vi "2 Think.vi"() -> ()   [LabVIEW 2011]
doc: "The Think VI performs the logic to determine which setpoints to send to the boat. Within the Think VI, a variety of systems take the boat information and output sail and rudder setpoints. The Think VI contains the arbiter VI which contains the logic used to determine which setpoints will ultimately be sent to the boat.\n\nWithin the Think VI, 5 systems are considered, in order of inherent priority:\n-Manual Override\n-Don't Flip\n-Staying out of/getting out of Irons\n-Getting to the goal\n-Default (such that there is always something being sent to the boat)"
uses:
  2 Globals/2 Global.vi
  2 Typedefs/sail setpt.ctl
  2 Typedefs/rudder angle.ctl
  2 Typedefs/setpoints to boat.ctl
  2 Typedefs/setpoints to arbiter.ctl
panel:
  out "Setpoints \nBefore Smoothing":T1
  out "Default Setpoints":T4
  out "Get to Goal Setpoints":T4
  out "Get Out of Irons Setpoints":T4
  out "Don't Flip Setpoints":T4
  out "Override Setpoints":T4
  out "Final Setpoints":T1
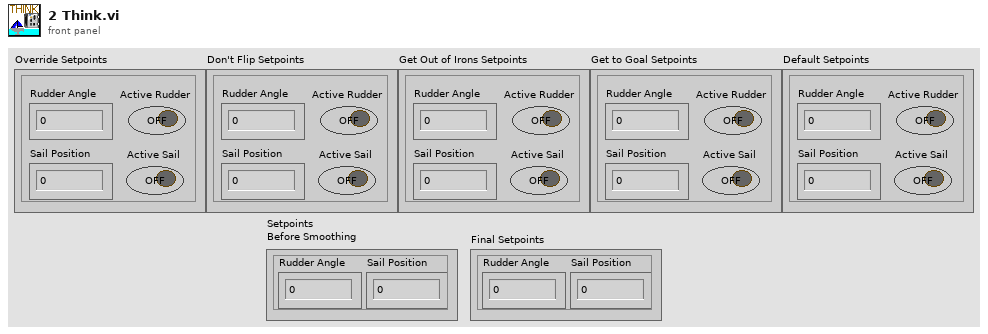
[diagram p1: front panel]
types:
  T1 = typedef "setpoints to boat.ctl" = cluster{"Sail Position":T2, "Rudder Angle":T3}
  T2 = typedef "sail setpt.ctl" = dbl
  T3 = typedef "rudder angle.ctl" = dbl
  T4 = typedef "setpoints to arbiter.ctl" = cluster{"Rudder Angle":dbl, "Sail Position":dbl, "Active Rudder":bool, "Active Sail":bool}
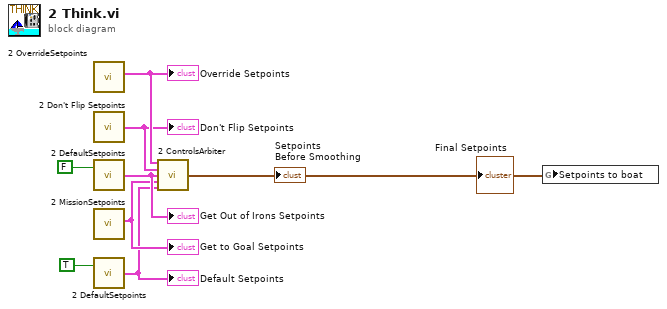
[diagram p0: block diagram]
diagram:
  n1 = call "2 OverrideSetpoints.vi"() -> ("Setpoints Out"=w8:T4)  [unwired: 11 in]
  "Override Setpoints" <- w8
  n2 = call "2 Don't Flip Setpoints.vi"() -> ("Setpoint Cluster"=w2:T4)  [unwired: 2 in]
  "Don't Flip Setpoints" <- w2
  n3 = call "2 DefaultSetpoints.vi"("Use Defaults"=FALSE) -> ("Setpoint Cluster"=w5:T4)  [unwired: 1 in]
  "Get Out of Irons Setpoints" <- w5
  n4 = call "2 MissionSetpoints.vi"() -> ("Setpoints Out"=w4:T4)  [unwired: 11 in]
  "Get to Goal Setpoints" <- w4
  n5 = call "2 DefaultSetpoints.vi"("Use Defaults"=TRUE) -> ("Setpoint Cluster"=w3:T4)  [unwired: 1 in]
  "Default Setpoints" <- w3
  n6 = call "2 ControlsArbiter.vi"("Manual Setpoints"=w8, "Dont Flip Setpoints"=w2, "Get out of Irons Setpoints"=w5, "Get to Goal Setpoints"=w4, "Default Setpoints"=w3) -> ("Final Setpoints"=w1:T1)  [unwired: 10 in]
  "Final Setpoints" <- w1
  "Setpoints \nBefore Smoothing" <- w1
  n7 = global write "2 Global.vi" "Setpoints to boat"(w1) -> ()
